vi "Async Console.vi"(0 "Console Listbox":refnum<vi>, 1 "Exit Event":refnum<user-event>, 5 "Full Command":string, 7 "Script Name":string, 9 "Log File":string, 11 "IP Address":string, 12 "Update Rate (ms)":i32) -> ()   [LabVIEW 2023]
uses:
  <vilib>/addons/_JKI Toolkits/State Machine/_JKI_lib_State_Machine.llb/Select State(s)_err__jki_lib_state_machine.vi
panel:
  out "standard error":string
  out "standard output":string
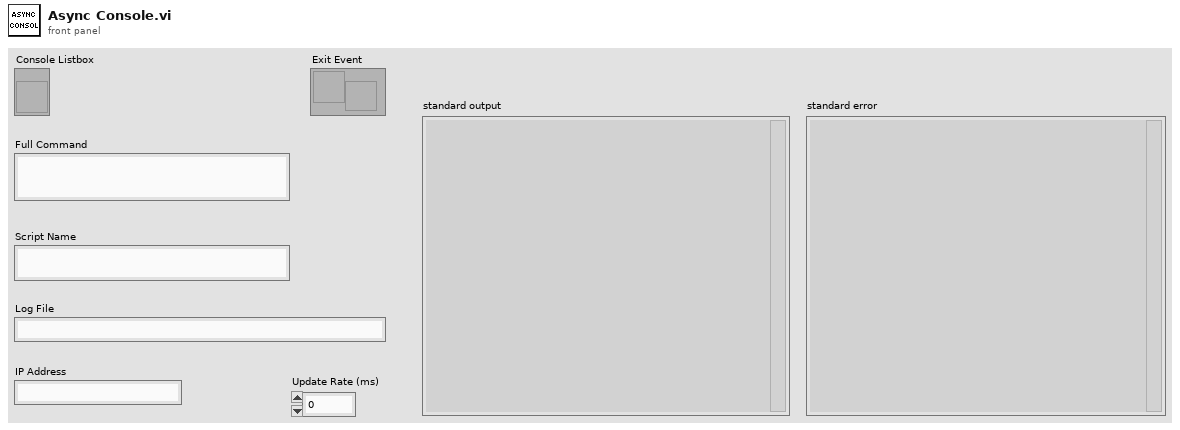
[diagram p1: front panel]
types:
  T1 = cluster{"Core":cluster{"Current VI Reference":refnum<vi>, "Close Panel on Exit?":bool}, "Process ID":i32}
  T2 = enum32{"Invalid", "Standard", "Closed", "Hidden", "Minimized", "Maximized"}
  T3 = enum32{"invalid app kind", "Development System", "Run Time System", "Student Edition", "Embedded LabVIEW", "Evaluation", "Custom"}
  T4 = cluster{"Current VI Reference":refnum<vi>, "Close Panel on Exit?":bool}
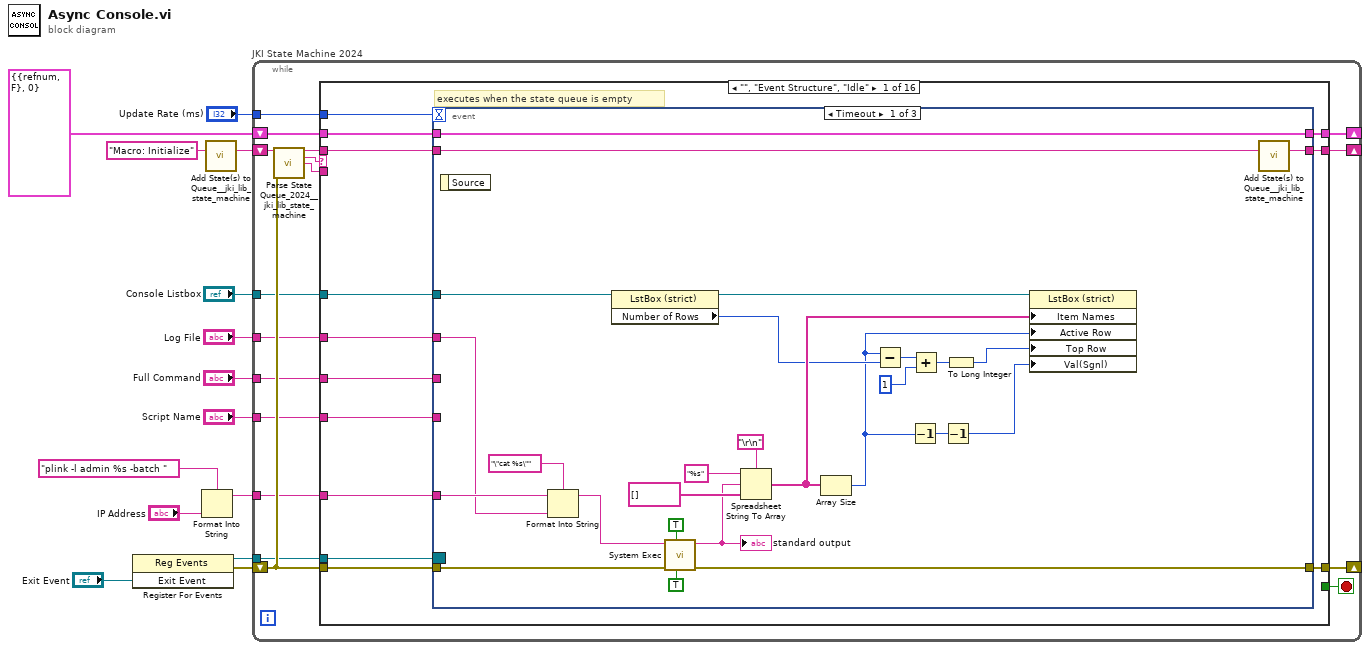
[diagram p0: block diagram]
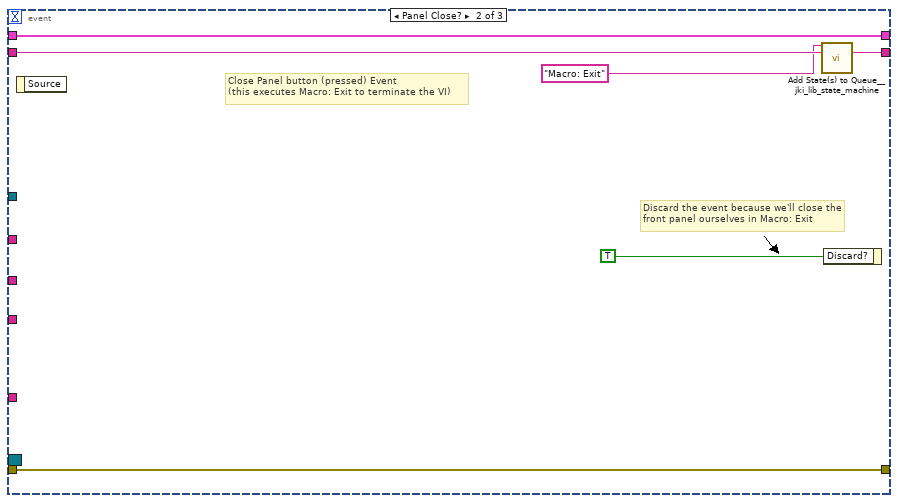
[diagram p2: hidden frame]
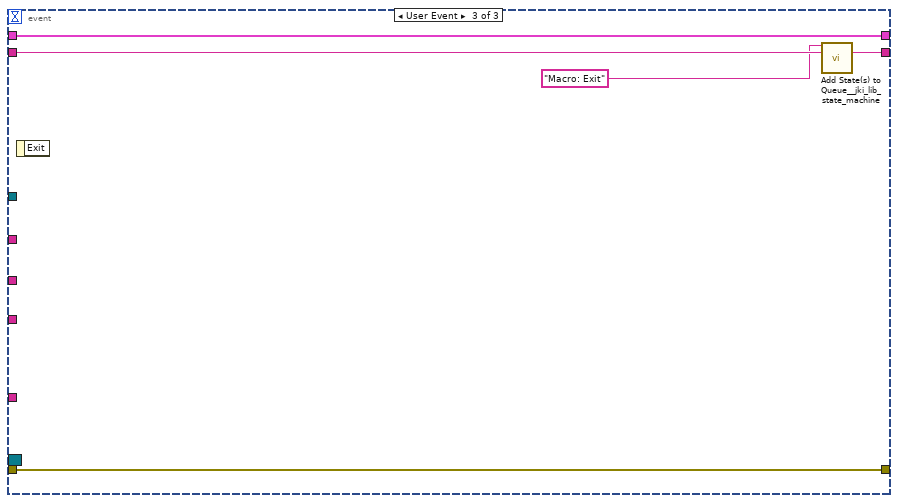
[diagram p3: hidden frame]
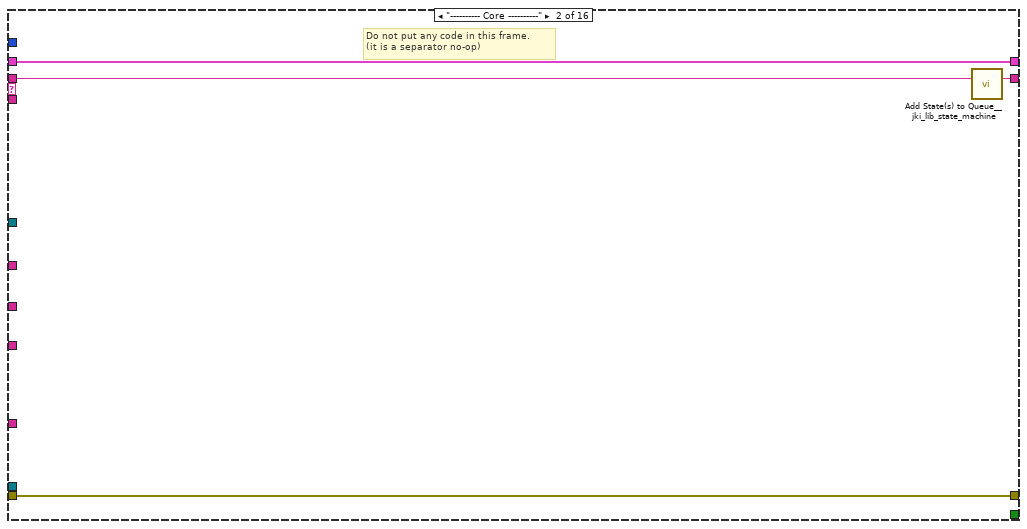
[diagram p4: hidden frame]
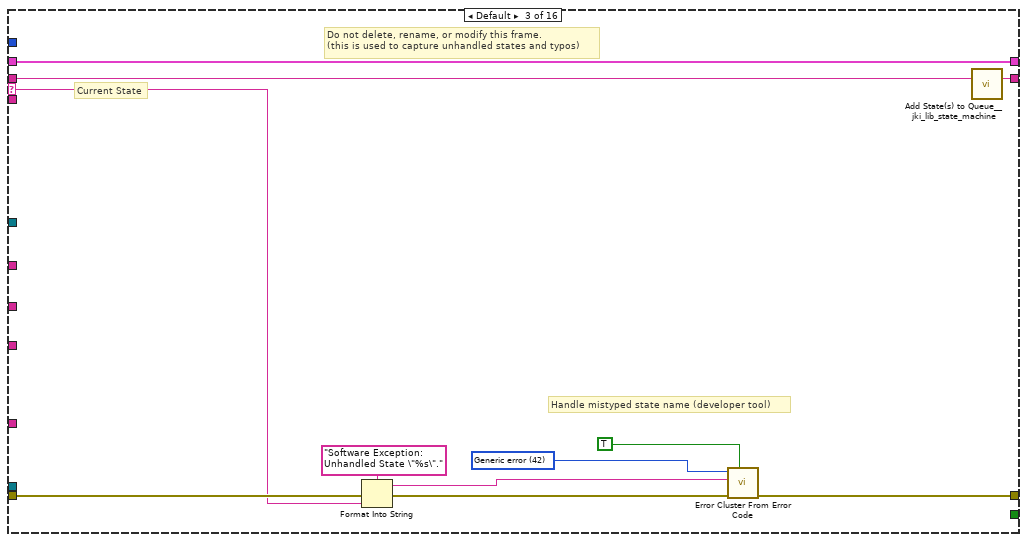
[diagram p5: hidden frame]
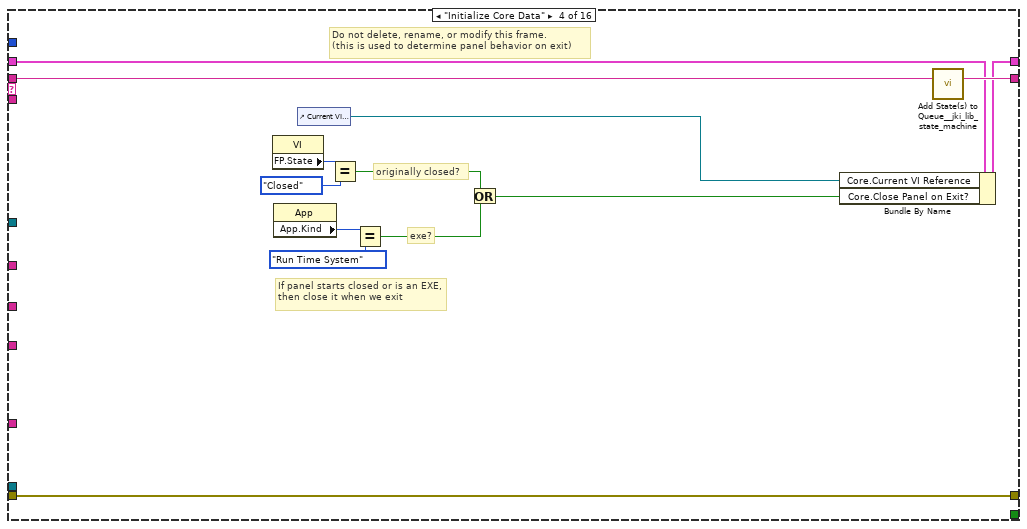
[diagram p6: hidden frame]
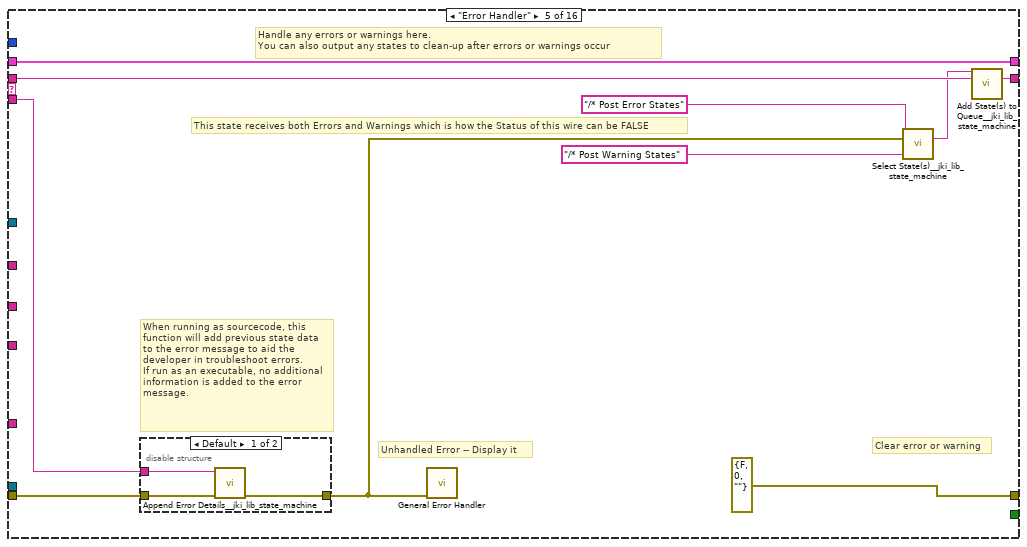
[diagram p7: hidden frame]
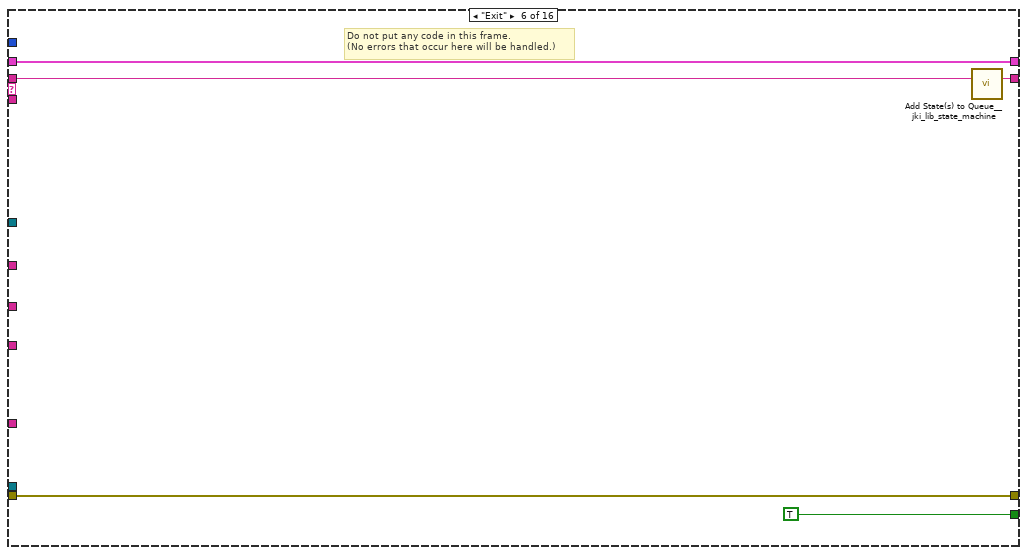
[diagram p9: hidden frame]
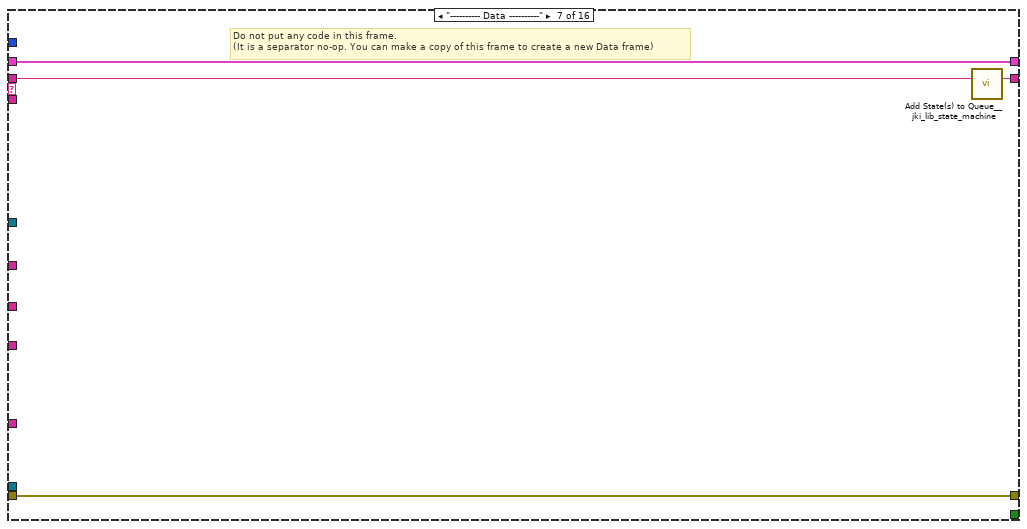
[diagram p10: hidden frame]
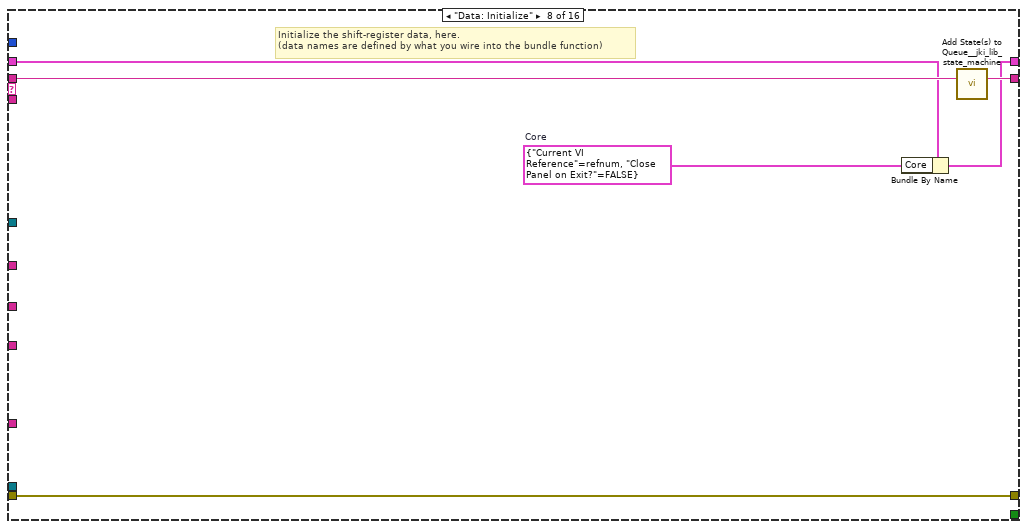
[diagram p11: hidden frame]
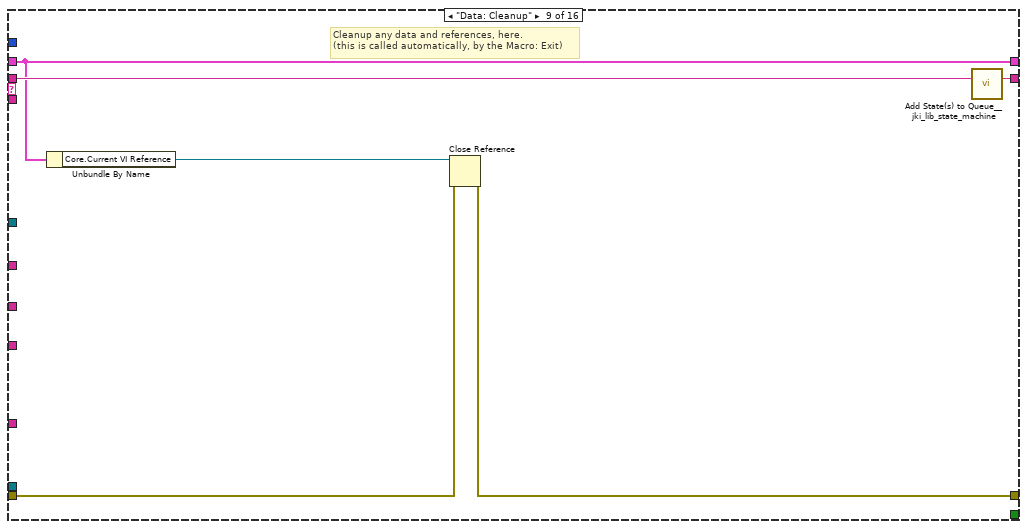
[diagram p12: hidden frame]
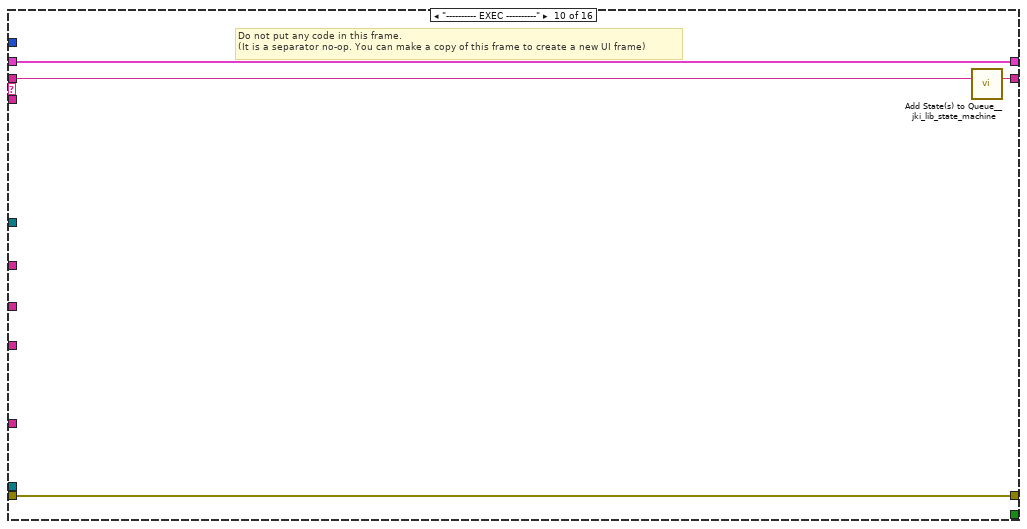
[diagram p13: hidden frame]
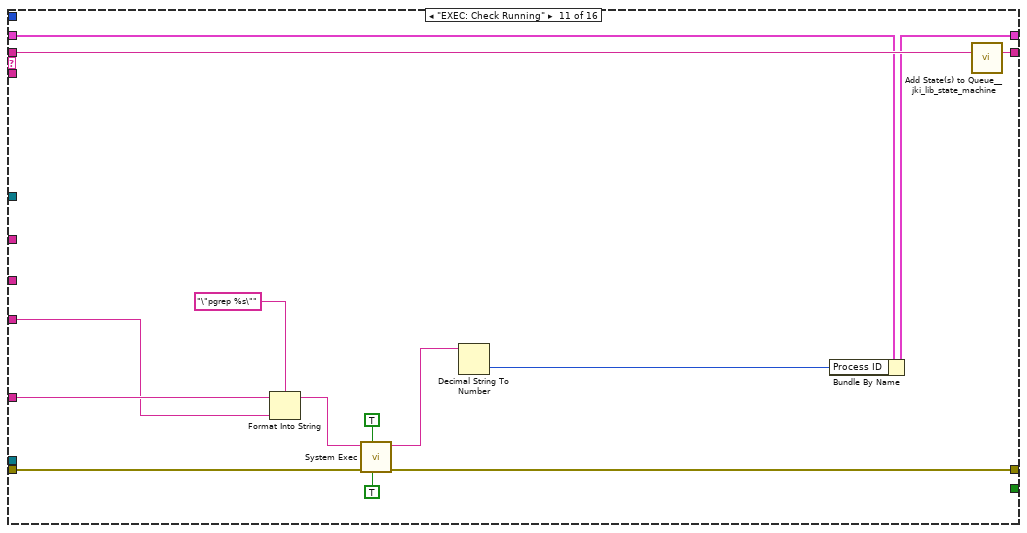
[diagram p14: hidden frame]
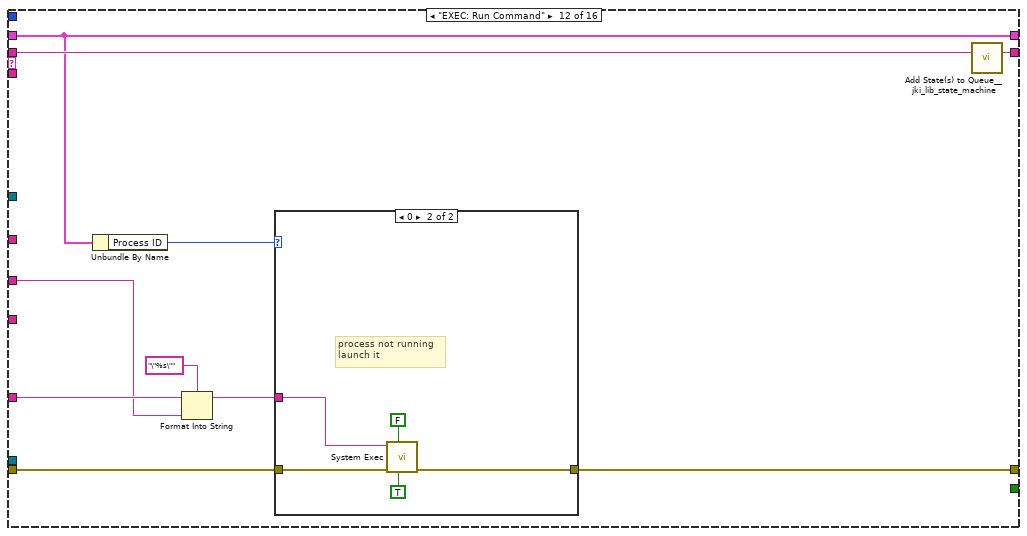
[diagram p15: hidden frame]
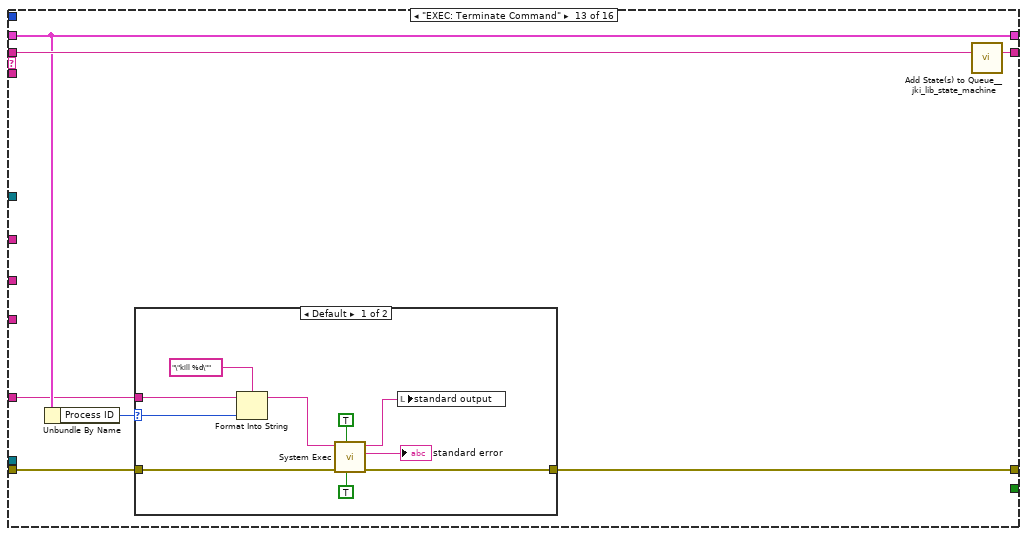
[diagram p17: hidden frame]
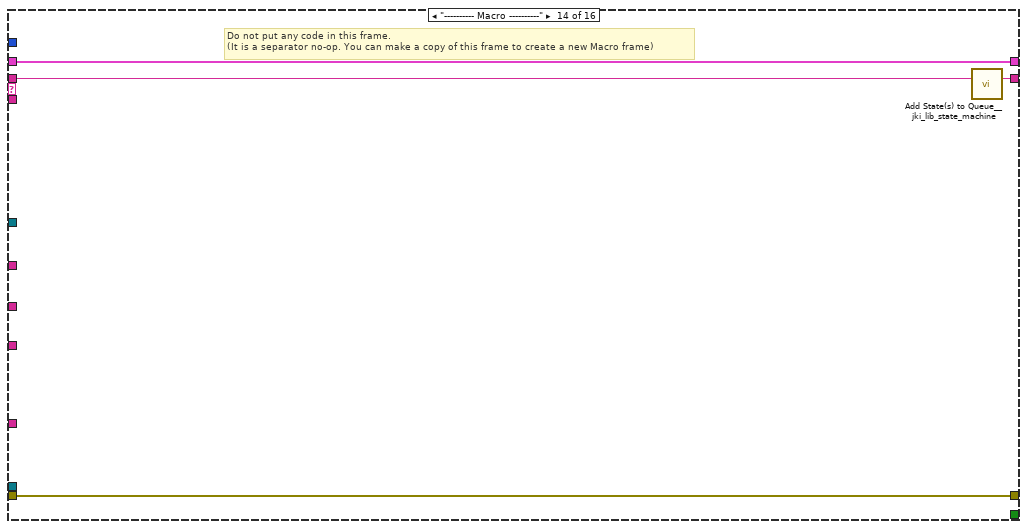
[diagram p19: hidden frame]
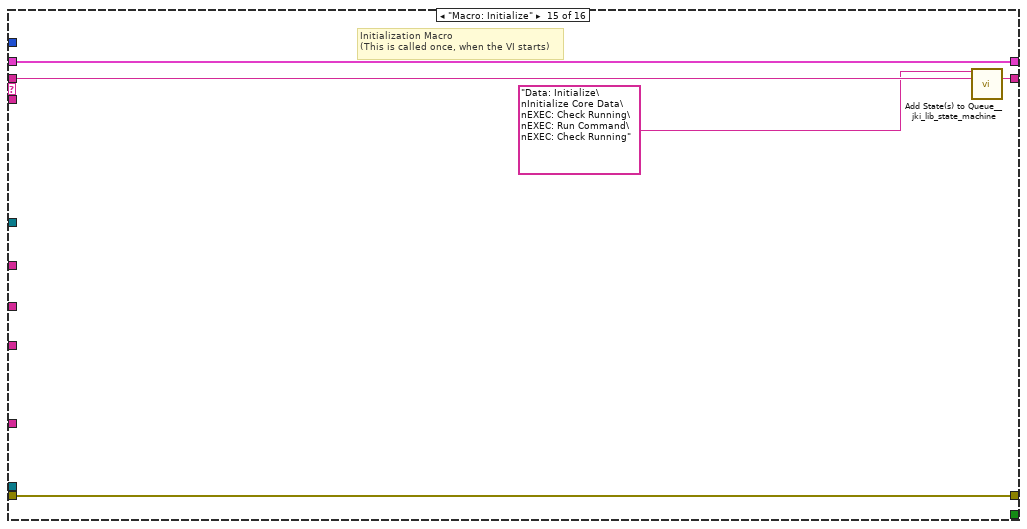
[diagram p20: hidden frame]
diagram:
  n1 = register-events("Exit Event") -> (reference out=w2:refnum<event-registration>, error out=w3:errorcluster)  [unwired: 2 in]
  n2 = Format Into String(format string="plink -l admin %s -batch ", "IP Address") -> (resulting string=w5:string)  [unwired: 2 in, 1 out]
  n3 = call <vilib>:"Add State(s) to Queue__jki_lib_state_machine.vi"("State(s) in (\"\")"="Macro: Initialize") -> ("States Out"=w14:string)  [unwired: 14 in]
  n4 = while "JKI State Machine 2024" {
    shift-right: [w24] -> _
    shift-left: T1 {"Core"={"Current VI Reference"=refnum, "Close Panel on Exit?"=FALSE}, "Process ID"=0} -> [w23]
    shift-right: [w27] -> _
    shift-left: w3 -> [w22]
    shift-right: [w26] -> _
    shift-left: w14 -> [w28]
    tunnel: "Update Rate (ms)" -> [w21]
    tunnel: "Full Command" -> [w20]
    tunnel: "Script Name" -> [w19]
    tunnel: "Console Listbox" -> [w18]
    tunnel: "Log File" -> [w17]
    tunnel: w5 -> [w16]
    tunnel: w2 -> [w15]
    stop <- w25 stop-if-true
    n5 = call <vilib>:"Parse State Queue_2024__jki_lib_state_machine.vi"("State Queue"=w28, "Error In (no error)"=w22) -> ("Remaining States"=w30:string, "Current State"=w31:string, "Arguments"=w29:string)  [unwired: 11 in]
    n6 = case shown="\"\", \"Event Structure\", \"Idle\"" w31 {
      selector: w31 -> [_ _ w86 _ _ _ _ _ _ _ _ _ _ _ _ _]
      tunnel: w30 -> [w44 w85 w90 w109 w119 w128 w132 w138 w144 w148 w162 w172 w185 w200 w205 w210]
      tunnel: w29 -> [_ _ _ _ w114 _ _ _ _ _ _ _ _ _ _ _]
      tunnel: w23 -> [w42 w82 w88 w102 w116 w126 w129 w135 w139 w145 w154 w168 w181 w197 w202 w208]
      tunnel: [w41 w83 w92 w106 errorcluster {"status"=FALSE, "code"=0, "source"=""} ("error out") w125 w130 w136 w140 w146 w151 w169 w182 w198 w203 w207] -> w27
      tunnel: w22 -> [w38 w83 w91 w106 w115 w125 w130 w136 w141 w146 w158 w170 w183 w198 w203 w207]
      tunnel: [w43 w84 w89 w108 w118 w127 w131 w137 w143 w147 w161 w171 w184 w199 w204 w209] -> w26
      tunnel: [_ _ _ _ _ TRUE _ _ _ _ _ _ _ _ _ _] -> w25
      tunnel: [w40 w82 w88 w107 w116 w126 w129 w133 w139 w145 w152 w168 w181 w197 w202 w208] -> w24
      tunnel: w21 -> [w39 _ _ _ _ _ _ _ _ _ _ _ _ _ _ _]
      tunnel: w20 -> [w37 _ _ _ _ _ _ _ _ _ _ w164 _ _ _ _]
      tunnel: w19 -> [w34 _ _ _ _ _ _ _ _ _ w149 _ _ _ _ _]
      tunnel: w18 -> [w36 _ _ _ _ _ _ _ _ _ _ _ _ _ _ _]
      tunnel: w17 -> [w35 _ _ _ _ _ _ _ _ _ _ _ _ _ _ _]
      tunnel: w16 -> [w33 _ _ _ _ _ _ _ _ _ w150 w166 w179 _ _ _]
      tunnel: w15 -> [w32 _ _ _ _ _ _ _ _ _ _ _ _ _ _ _]
      frame "", "Event Structure", "Idle" {
        # "executes when the state queue is empty"
        n7 = event shown="[0] Timeout" {
          selector: w32 -> [_ _ _]
          dyn-events: _ -> [_ _ _]
          timeout: w39 -> [_ _ _]
          tunnel: w44 -> [w70 w76 w79]
          tunnel: [w69 w75 w77] -> w43
          tunnel: w42 -> [w68 w73 w81]
          tunnel: [w64 w74 w80] -> w41
          tunnel: w38 -> [w65 w74 w80]
          tunnel: [w68 w73 w81] -> w40
          tunnel: w37 -> [_ _ _]
          tunnel: w36 -> [w55 _ _]
          tunnel: w35 -> [w61 _ _]
          tunnel: w34 -> [_ _ _]
          tunnel: w33 -> [w63 _ _]
          event Timeout {
            n8 = event-data() -> ()  [unwired: 1 in, 1 out]
            n9 = Format Into String(format string="\"cat %s\"", initial string=w63, w61) -> (resulting string=w60:string)  [unwired: 1 in, 1 out]
            n10 = property class="LstBox (strict)"(reference=w55) -> (reference out=w54:refnum<vi>, "Number of Rows"=w48:u32)  [unwired: 1 in, 1 out]
            n11 = call <vilib>:"System Exec.vi"("run minimized? (F)"=TRUE, "wait until completion? (T)"=TRUE, "error in (no error)"=w65, "command line"=w60) -> ("error out"=w64:errorcluster, "standard output"=w58:string)  [unwired: 4 in, 2 out]
            "standard output" <- w58
            n12 = Spreadsheet String To Array(delimiter (Tab)="\r\n", format string="%s", spreadsheet string=w58, array type (2D Dbl)=string[] []) -> (array=w49:string[])
            n13 = Array Size(array=w49) -> (size(s)=w46:i32)
            n14 = Subtract(x=w46, y=w48) -> (x-y=w53:u32)
            n15 = Decrement(x=w46) -> (x-1=w45:i32)
            n16 = Add(x=w53, y=u32 1) -> (x+y=w51:u32)
            n17 = Decrement(x=w45) -> (x-1=w47:i32)
            n18 = To Long Integer(number=w51) -> (32bit integer=w50:i32)
            n19 = property class="LstBox (strict)"(reference=w54, "Item Names"=w49, "Active Row"=w46, "Top Row"=w50, "Val(Sgnl)"=w47) -> ()  [unwired: 1 in, 2 out]
            n20 = call <vilib>:"Add State(s) to Queue__jki_lib_state_machine.vi"("State(s) in (\"\")"=w70) -> ("States Out"=w69:string)  [unwired: 14 in]
          }
          event Panel Close? {
            # "Discard the event because we'll close the front panel ourselves in Macro: Exit"
            # "Close Panel button (pressed) Event\n(this executes Macro: Exit to terminate the VI)"
            n21 = event-data() -> ()  [unwired: 1 in, 1 out]
            n22 = call <vilib>:"Add State(s) to Queue__jki_lib_state_machine.vi"("State(s) in Front (\"\")"="Macro: Exit", "State(s) in (\"\")"=w76) -> ("States Out"=w75:string)  [unwired: 13 in]
            n23 = event-data("Discard?"=TRUE) -> ()  [unwired: 1 in, 1 out]
          }
          event User Event {
            n24 = event-data() -> ()  [unwired: 1 in, 1 out]
            n25 = call <vilib>:"Add State(s) to Queue__jki_lib_state_machine.vi"("State(s) in Front (\"\")"="Macro: Exit", "State(s) in (\"\")"=w79) -> ("States Out"=w77:string)  [unwired: 13 in]
          }
        }
      }
      frame "---------- Core ----------" {
        # "Do not put any code in this frame.\n(it is a separator no-op)"
        n26 = call <vilib>:"Add State(s) to Queue__jki_lib_state_machine.vi"("State(s) in (\"\")"=w85) -> ("States Out"=w84:string)  [unwired: 14 in]
      }
      frame Default {
        w95 = 42 items=["No error", "Argument error", "Memory is full", "Out of zone", "End of file", "File already open", "Generic file I/O error", "File not found", "File permission error", "Disk is full", "Duplicate path", "Too many files open", "System feature not enabled", "Resource file not found", "Cannot add resource", "Resource not found", "Image not found", "Image memory error", "Pen does not exist", "Config type invalid", "Config token not found", "Config parse error", "Config memory error", "Bad external code format", "Bad external code offset", "External code not present", "Null window", "Destroy window error", "Null menu", "Print aborted", "Bad print record", "Print driver error", "Windows error during printing", "Memory error during printing", "Print dialog error", "Generic print error", "Invalid device refnum", "Device not found", "Device parameter error", "Device unit error", "Cannot open device", "Device call aborted", "Generic error", "Cancelled by user", "Object ID too low", "Object ID too high", "Object not in heap", "Unknown heap", "Unknown object (invalid DefProc)", "Unknown object (DefProc not in table)", "Message out of range", "Invalid (null) method", "Unknown message", "Manager call not supported", "Bad address", "Network operation in progress", "Network operation timed out", "Connection is busy", "Network attribute not supported", "Network error", "Address in use", "System out of memory", "Connection aborted", "Connection refused", "Not connected", "Already connected", "Connection closed", "Initialization error (interapplication manager)", "Bad occurrence", "Wait on unbound occurrence handler", "Occurrence queue overflow", "Datalog type conflict", "Unused", "Unrecognized type (interapplication manager)", "Memory corrupt", "Failed to make temporary DLL", "Old CIN version", "Drag socket not found", "Failed to load drop-object", "Failed to register OLE object", "Failed to release OLE object", "Format specifier type mismatch", "Unknown format specifier", "Too few format specifiers", "Too many format specifiers", "Scan failed", "Newer CIN version", "Error converting to variant", "Runtime menu error", "Password tampered", "Variant attribute not found", "Incompatible variant data type", "Event data is not available", "Event Store is not present", "Occurrence is not found", "Event Queue is not created", "Event info is not available", "Refnum passed is NULL", "Error retrieving Class GUID", "Error retrieving CoClass GUID", "Error retrieving TypeLib GUID.", "Bad built application magic bytes.", "Specific driver is different from the specific driver associated with the Logical Name.", "There is no session opened to the class driver.", "Max Error", "MAX - Error with config objects", "MAX - Error loading configuration", "MAX - Group not supported"]
        # "Current State"
        # "Do not delete, rename, or modify this frame.\n(this is used to capture unhandled states and typos)"
        # "Handle mistyped state name (developer tool)"
        n27 = Format Into String(format string="Software Exception: Unhandled State \"%s\"." ("message"), error in=w91, w86) -> (resulting string=w94:string, error out=w93:errorcluster)  [unwired: 1 in]
        n28 = call <vilib>:"Error Cluster From Error Code.vi"("show call chain? (False)"=TRUE, "error in (no error)"=w93, "error message (\"\")"=w94, "error code (0)"=w95) -> ("error out"=w92:errorcluster)  [unwired: 5 in]
        n29 = call <vilib>:"Add State(s) to Queue__jki_lib_state_machine.vi"("State(s) in (\"\")"=w90) -> ("States Out"=w89:string)  [unwired: 14 in]
      }
      frame "Initialize Core Data" {
        # "Do not delete, rename, or modify this frame.\n(this is used to determine panel behavior on exit)"
        # "originally closed?"
        # "exe?"
        # "If panel starts closed or is an EXE, then close it when we exit"
        n30 = property class="VI"() -> ("FP.State"=w99:T2)  [unwired: 2 in, 2 out]
        n31 = property class="App"() -> ("App.Kind"=w105:T3)  [unwired: 2 in, 2 out]
        n32 = control-ref of="Current VI Reference"() -> (w100:refnum<vi>)
        n33 = Equal?(x=w99, y=T2."Closed" ("Front Panel Window:State")) -> (x = y?=w97:bool)
        n34 = Equal?(x=w105, y=T3."Run Time System" ("Application:Kind")) -> (x = y?=w103:bool)
        n35 = Or(x=w97, y=w103) -> (x .or. y?=w101:bool)
        n36 = Bundle By Name(cluster=w102, "Core.Current VI Reference"=w100, "Core.Close Panel on Exit?"=w101) -> (w107:T1)
        n37 = call <vilib>:"Add State(s) to Queue__jki_lib_state_machine.vi"("State(s) in (\"\")"=w109) -> ("States Out"=w108:string)  [unwired: 14 in]
      }
      frame "Error Handler" {
        # "When running as sourcecode, this function will add previous state data to the error message to aid the developer in troubleshoot errors.\nIf run as an executable, no additional information is added to the error message."
        # "This state receives both Errors and Warnings which is how the Status of this wire can be FALSE"
        # "Unhandled Error -- Display it"
        # "Handle any errors or warnings here.\nYou can also output any states to clean-up after errors or warnings occur"
        # "Clear error or warning"
        n38 = disable-structure shown="Default" {
          disable-tunnel: w115 -> [w122 w123]
          disable-tunnel: w114 -> [w121 _]
          disable-tunnel: [w120 w123] -> w113
          frame condition #0 (active) {
            n39 = call <vilib>:"Append Error Details__jki_lib_state_machine.vi"("error in (no error)"=w122, "Previous State and Argument(s)"=w121) -> ("error out"=w120:errorcluster)  [unwired: 9 in]
          }
          frame condition #1 {
          }
        }
        n40 = call <vilib>:"General Error Handler.vi"("error in (no error)"=w113) -> ()  [unwired: 10 in, 5 out]
        n41 = call-poly <vilib>:"Select State(s)__jki_lib_state_machine.vi"("State(s) if True (\"\")"="/* Post Error States", "Select"=w113, "State(s) if False (\"\")"="/* Post Warning States") -> ("States Out"=w111:string)  [unwired: 12 in]
        n42 = call <vilib>:"Add State(s) to Queue__jki_lib_state_machine.vi"("State(s) in Front (\"\")"=w111, "State(s) in (\"\")"=w119) -> ("States Out"=w118:string)  [unwired: 13 in]
      }
      frame "Exit" {
        # "Do not put any code in this frame.\n(No errors that occur here will be handled.)"
        n43 = call <vilib>:"Add State(s) to Queue__jki_lib_state_machine.vi"("State(s) in (\"\")"=w128) -> ("States Out"=w127:string)  [unwired: 14 in]
      }
      frame "---------- Data ----------" {
        # "Do not put any code in this frame.\n(It is a separator no-op. You can make a copy of this frame to create a new Data frame)"
        n44 = call <vilib>:"Add State(s) to Queue__jki_lib_state_machine.vi"("State(s) in (\"\")"=w132) -> ("States Out"=w131:string)  [unwired: 14 in]
      }
      frame "Data: Initialize" {
        w134 = T4 {"Current VI Reference"=refnum, "Close Panel on Exit?"=FALSE}  # Core
        # "Initialize the shift-register data, here.\n(data names are defined by what you wire into the bundle function)"
        n45 = Bundle By Name(cluster=w135, "Core"=w134) -> (w133:T1)
        n46 = call <vilib>:"Add State(s) to Queue__jki_lib_state_machine.vi"("State(s) in (\"\")"=w138) -> ("States Out"=w137:string)  [unwired: 14 in]
      }
      frame "Data: Cleanup" {
        # "Cleanup any data and references, here.\n(this is called automatically, by the Macro: Exit)"
        n47 = Unbundle By Name(w139) -> ("Core.Current VI Reference"=w142:refnum<vi>)
        n48 = Close Reference(reference=w142, error in (no error)=w141) -> (error out=w140:errorcluster)
        n49 = call <vilib>:"Add State(s) to Queue__jki_lib_state_machine.vi"("State(s) in (\"\")"=w144) -> ("States Out"=w143:string)  [unwired: 14 in]
      }
      frame "---------- EXEC ----------" {
        # "Do not put any code in this frame.\n(It is a separator no-op. You can make a copy of this frame to create a new UI frame)"
        n50 = call <vilib>:"Add State(s) to Queue__jki_lib_state_machine.vi"("State(s) in (\"\")"=w148) -> ("States Out"=w147:string)  [unwired: 14 in]
      }
      frame "EXEC: Check Running" {
        n51 = Format Into String(format string="\"pgrep %s\"", initial string=w150, w149) -> (resulting string=w156:string)  [unwired: 1 in, 1 out]
        n52 = call <vilib>:"System Exec.vi"("run minimized? (F)"=TRUE, "wait until completion? (T)"=TRUE, "error in (no error)"=w158, "command line"=w156) -> ("error out"=w151:errorcluster, "standard output"=w155:string)  [unwired: 4 in, 2 out]
        n53 = Decimal String To Number(string=w155) -> (number=w153:i32)  [unwired: 2 in, 1 out]
        n54 = Bundle By Name(cluster=w154, "Process ID"=w153) -> (w152:T1)
        n55 = call <vilib>:"Add State(s) to Queue__jki_lib_state_machine.vi"("State(s) in (\"\")"=w162) -> ("States Out"=w161:string)  [unwired: 14 in]
      }
      frame "EXEC: Run Command" {
        n56 = Unbundle By Name(w168) -> ("Process ID"=w167:i32)
        n57 = Format Into String(format string="\"%s\"", initial string=w166, w164) -> (resulting string=w163:string)  [unwired: 1 in, 1 out]
        n58 = case shown="0" w167 {
          tunnel: w170 -> [w173 w176]
          tunnel: [w173 w175] -> w169
          tunnel: w163 -> [_ w174]
          frame Default {
            # "process already running\ndont launch again"
          }
          frame 0 {
            # "process not running\nlaunch it"
            n59 = call <vilib>:"System Exec.vi"("run minimized? (F)"=TRUE, "wait until completion? (T)"=FALSE, "error in (no error)"=w176, "command line"=w174) -> ("error out"=w175:errorcluster)  [unwired: 4 in, 3 out]
          }
        }
        n60 = call <vilib>:"Add State(s) to Queue__jki_lib_state_machine.vi"("State(s) in (\"\")"=w172) -> ("States Out"=w171:string)  [unwired: 14 in]
      }
      frame "EXEC: Terminate Command" {
        n61 = Unbundle By Name(w181) -> ("Process ID"=w180:i32)
        n62 = case shown="Default" w180 {
          selector: w180 -> [w190 _]
          tunnel: w183 -> [w193 w196]
          tunnel: [w192 w196] -> w182
          tunnel: w179 -> [w186 _]
          frame Default {
            n63 = Format Into String(format string="\"kill %d\"", initial string=w186, w190) -> (resulting string=w189:string)  [unwired: 1 in, 1 out]
            n64 = call <vilib>:"System Exec.vi"("run minimized? (F)"=TRUE, "wait until completion? (T)"=TRUE, "error in (no error)"=w193, "command line"=w189) -> ("error out"=w192:errorcluster, "standard error"=→"standard error":string, "standard output"=w188:string)  [unwired: 4 in, 1 out]
            n65 = local write "standard output"(w188) -> ()
          }
          frame 0 {
            # "process not running\nnothing to terminate"
          }
        }
        n66 = call <vilib>:"Add State(s) to Queue__jki_lib_state_machine.vi"("State(s) in (\"\")"=w185) -> ("States Out"=w184:string)  [unwired: 14 in]
      }
      frame "---------- Macro ----------" {
        # "Do not put any code in this frame.\n(It is a separator no-op. You can make a copy of this frame to create a new Macro frame)"
        n67 = call <vilib>:"Add State(s) to Queue__jki_lib_state_machine.vi"("State(s) in (\"\")"=w200) -> ("States Out"=w199:string)  [unwired: 14 in]
      }
      frame "Macro: Initialize" {
        # "Initialization Macro\n(This is called once, when the VI starts)"
        n68 = call <vilib>:"Add State(s) to Queue__jki_lib_state_machine.vi"("State(s) in Front (\"\")"="Data: Initialize\nInitialize Core Data\nEXEC: Check Running\nEXEC: Run Command\nEXEC: Check Running", "State(s) in (\"\")"=w205) -> ("States Out"=w204:string)  [unwired: 13 in]
      }
      frame "Macro: Exit" {
        # "Exit Macro\n(This is called once, when the VI exits)"
        n69 = call <vilib>:"Add State(s) to Queue__jki_lib_state_machine.vi"("State(s) in Front (\"\")"="EXEC: Terminate Command\nData: Cleanup\nExit", "State(s) in (\"\")"=w210) -> ("States Out"=w209:string)  [unwired: 13 in]
      }
    }
  }
